vi "report_view.vi"   [LabVIEW 2025]
doc: "VI para poder visualizar Reportes TDMS \nSe debe llamar desde un VI principal o abrir este mismo VI y darle play \nSe abrira una ventana de dialogo para seleccionar el reporte"
uses:
  <vilib>/Utility/TDMS File Viewer/NI_TDMS File Viewer.lvlib
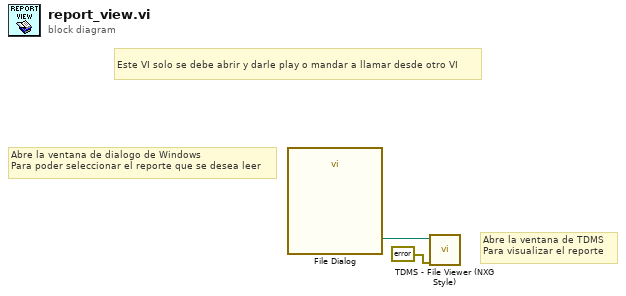
[diagram p0: block diagram]
diagram:
  # "Este VI solo se debe abrir y darle play o mandar a llamar desde otro VI"
  # "Abre la ventana de TDMS\nPara visualizar el reporte"
  # "Abre la ventana de dialogo de Windows\nPara poder seleccionar el reporte que se desea leer"
  n1 = call "File Dialog"() -> ("selected path"=w2:path)  [unwired: 12 in, 3 out]
  n2 = call <vilib>:"TDMS - File Viewer (NXG Style).vi"("error in"=errorcluster {"status"=FALSE, "code"=0, "source"=""}, "file in"=w2) -> ()  [unwired: 8 in, 2 out]
